vi "ExampleBotsDirectory.vi"() -> (3 "stripped path":path)   [LabVIEW 2015]
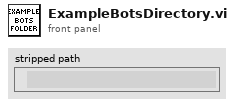
[diagram p1: front panel]
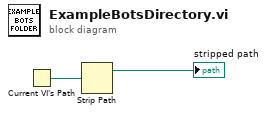
[diagram p0: block diagram]
diagram:
  n1 = Current VI's Path() -> (path=w2:path)
  n2 = Strip Path(path=w2) -> (stripped path=→"stripped path":path)  [unwired: 1 out]
